vi "Write Document Source.vi"(8 "error in (no error)":errorcluster, 10 "Value":string, 11 "WebView2 Control in":refnum<class "WebView2 Control.lvclass">) -> (0 "error out":errorcluster, 3 "WebView2 Control out":refnum<class "WebView2 Control.lvclass">)   [LabVIEW 2020, in "WebView2.lvlib" / "WebView2 Control.lvclass"]
uses:
  WebView2 Control.lvclass
  WebView2 Control.lvclass/WebView2 Control.ctl
  C:/Users/Simon/Documents/GitHub/LV-WebView2/Source/Libs/Microsoft.Web.WebView2.Core.dll
  Libs/Microsoft.Web.WebView2.Core.dll
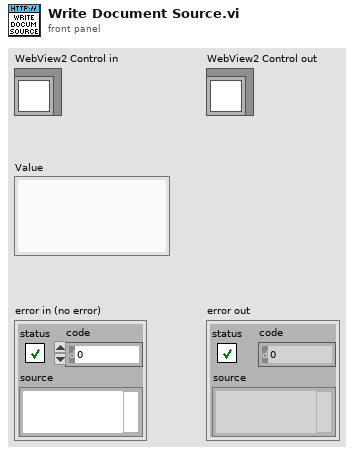
[diagram p1: front panel]
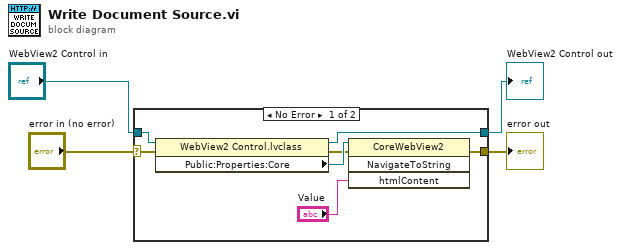
[diagram p0: block diagram]
diagram:
  n1 = case shown="No Error" "error in (no error)" {
    selector: "error in (no error)" -> [w9 w13]
    tunnel: "WebView2 Control in" -> [w7 w12]
    tunnel: [w11 w13] -> w1
    tunnel: [w8 w12] -> w3
    frame No Error {
      n2 = property class="WebView2 Control.lvclass"(reference=w7, error in=w9) -> (reference out=w8:refnum<class "WebView2 Control.lvclass">, error out=w5:errorcluster, "Public:Properties:Core"=w6:refnum<k24>)
      n3 = invoke class="CoreWebView2" method="NavigateToString"(reference=w6, error in=w5, "htmlContent"="Value") -> (error out=w11:errorcluster)  [unwired: 1 in, 3 out]
    }
    frame Error {
    }
  }
  "error out" <- w1
  "WebView2 Control out" <- w3
